vi "setGyroODR.vi"() -> ()   [LabVIEW 2016]
uses:
  #defines.ctl
  GLOBALS.vi
panel:
  in  "gRate":u8
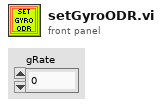
[diagram p1: front panel]
types:
  T1 = typedef "#defines.ctl" = i8
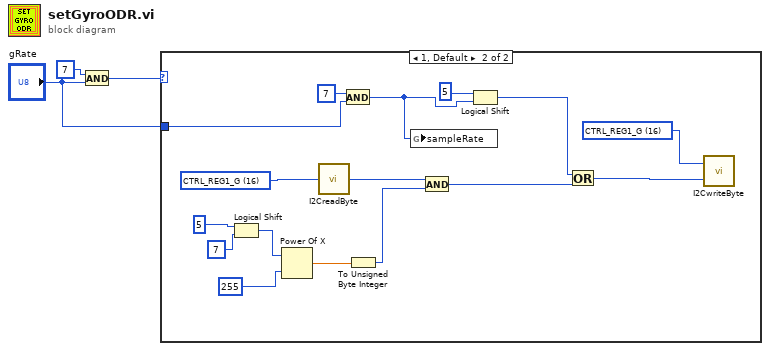
[diagram p0: block diagram]
diagram:
  n1 = And(x=u8 7, y="gRate") -> (x .and. y?=w2:u8)
  n2 = case shown="1, Default" w2 {
    tunnel: "gRate" -> [_ w10]
    frame 0 {
    }
    frame 1, Default {
      w4 = T1 16 items=["CTRL_REG9_G"=35, "STATUS_REG_1"=39, "OUT_X_L_XL"=40, "FIFO_CTRL"=46, "FIFO_SRC"=47, "CTRL_REG4_G"=30, "OUT_X_L_G"=24, "OUT_TEMP_L"=21, "INT_GEN_SRC_G"=20, "ORIENT_CFG_G"=19, "CTRL_REG3_G"=18, "CTRL_REG2_G"=17, "CTRL_REG1_G"=16, "WHO_AM_I_XG"=15] ("Ring")
      w19 = T1 16 items=["CTRL_REG9_G"=35, "STATUS_REG_1"=39, "OUT_X_L_XL"=40, "FIFO_CTRL"=46, "FIFO_SRC"=47, "CTRL_REG4_G"=30, "OUT_X_L_G"=24, "OUT_TEMP_L"=21, "INT_GEN_SRC_G"=20, "ORIENT_CFG_G"=19, "CTRL_REG3_G"=18, "CTRL_REG2_G"=17, "CTRL_REG1_G"=16, "WHO_AM_I_XG"=15] ("Ring")
      n3 = Logical Shift(y=i16 5, x=u8 7) -> (x << y=w14:u8)
      n4 = Power Of X(1:u8 255 ("x"), 2:w14) -> (0:w13:dbl)
      n5 = call "I2CreadByte.vi"("subAddress"=w19) -> ("data"=w18:u8)
      n6 = And(x=u8 7, y=w10) -> (x .and. y?=w6:u8)
      n7 = To Unsigned Byte Integer(number=w13) -> (unsigned 8bit integer=w12:u8)
      n8 = global write "GLOBALS.vi" "sampleRate"(w6) -> ()
      n9 = And(x=w18, y=w12) -> (x .and. y?=w11:u8)
      n10 = Logical Shift(y=i16 5, x=w6) -> (x << y=w7:u8)
      n11 = Or(x=w7, y=w11) -> (x .or. y?=w5:u8)
      n12 = call "I2CwriteByte.vi"("data"=w5, "subAddress"=w4) -> ()  [unwired: 1 in]
    }
  }
